vi "CreatFoldeFile.vi"(8 "error in":errorcluster, 11 "Path":path=path "D:/全域高斯機 參數/Data") -> (0 "error out":errorcluster, 2 "fileExist?":bool, 3 "path":path)   [LabVIEW 2015]
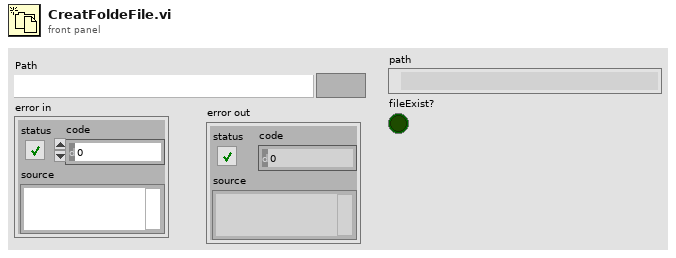
[diagram p1: front panel]
types:
  T1 = enum16{"open", "replace", "create", "open or create", "replace or create", "replace or create with confirmation"}
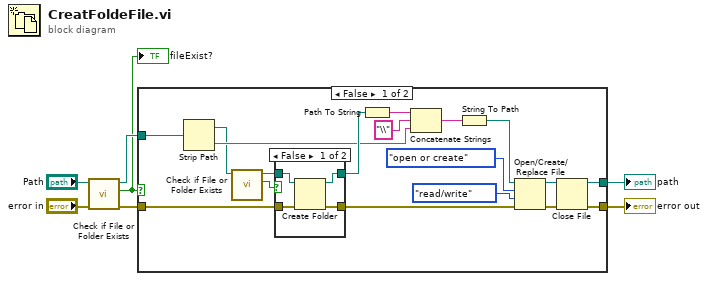
[diagram p0: block diagram]
diagram:
  n1 = call <vilib>:"Check if File or Folder Exists.vi"("error in (no error)"="error in", "path"="Path") -> ("error out"=w5:errorcluster, "file or folder exists?"=w1:bool, "dup path"=w6:path)  [unwired: 7 in]
  "fileExist?" <- w1
  n2 = case shown="False" w1 {
    tunnel: w6 -> [w25 w33]
    tunnel: w5 -> [w18 w32]
    tunnel: [w13 w33] -> w4
    tunnel: [w15 w32] -> w2
    frame False {
      n3 = Strip Path(path=w25) -> (stripped path=w9:path, name=w21:string)
      n4 = call <vilib>:"Check if File or Folder Exists.vi"("path"=w9) -> ("file or folder exists?"=w10:bool, "dup path"=w8:path)  [unwired: 8 in, 1 out]
      n5 = case shown="False" w10 {
        tunnel: [w28 w30] -> w24
        tunnel: w18 -> [w27 w31]
        tunnel: [w26 w31] -> w11
        tunnel: w8 -> [w29 w30]
        frame False {
          n6 = Create Folder(path (use dialog)=w29, error in=w27) -> (created path=w28:path, error out=w26:errorcluster)  [unwired: 1 in, 1 out]
        }
        frame True {
        }
      }
      n7 = Path To String(path=w24) -> (string=w23:string)
      n8 = Concatenate Strings(w23, "\\" ("string"), w21) -> (w20:string)
      n9 = String To Path(string=w20) -> (path=w14:path)
      n10 = Open/Create/Replace File(file path (use dialog)=w14, error in=w11, operation (0:open)=T1."open or create", access (0:read/write)=enum16{"read/write", "read-only", "write-only"}."read/write") -> (refnum out=w17:refnum<file>, error out=w16:errorcluster)  [unwired: 2 in, 1 out]
      n11 = Close File(refnum=w17, error in=w16) -> (path=w13:path, error out=w15:errorcluster)
    }
    frame True {
    }
  }
  "path" <- w4
  "error out" <- w2
